vi "클러스터.vi"() -> ()   [LabVIEW 2014]
panel:
  out "클러스터 4":T1
  in  "클러스터 3":T1={"숫자형"=4.12, "확인 버튼"=TRUE, "문자열"="hello", "배열"=[1.0, -2.0, 3.0, -3.0, 7.5], "error in (no error)"={"status"=FALSE, "code"=0, "source"=""}}
  out "클러스터 2":T1
  in  "클러스터":T1={"숫자형"=4.12, "확인 버튼"=TRUE, "문자열"="hello", "배열"=[1.0, -2.0, 3.0, -3.0, 7.5], "error in (no error)"={"status"=FALSE, "code"=0, "source"=""}}
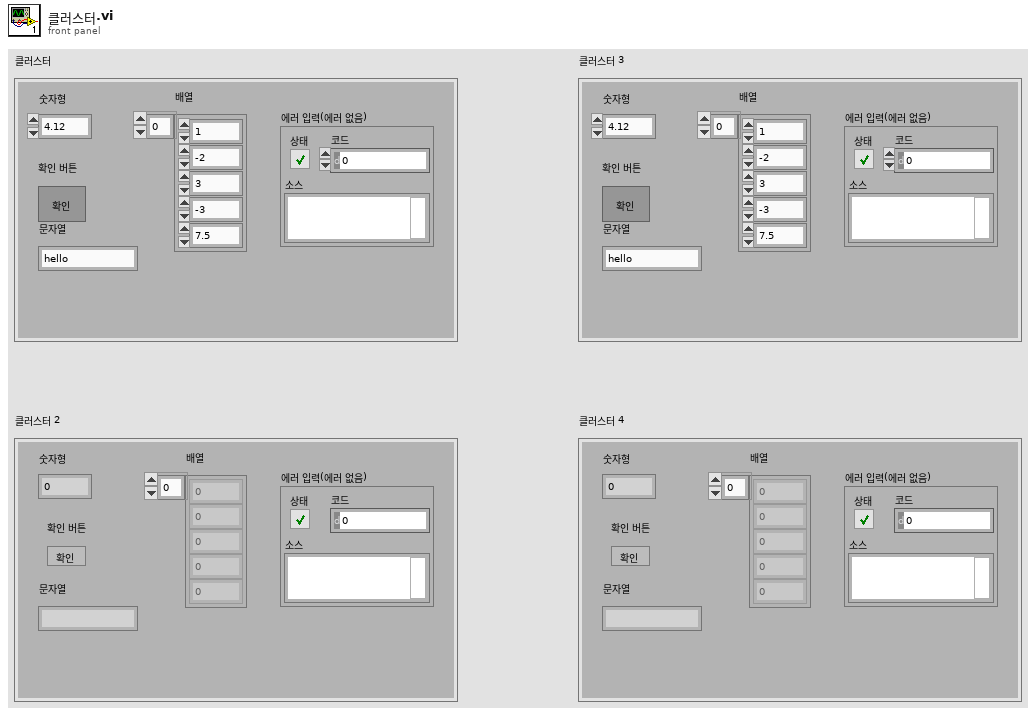
[diagram p1: front panel]
types:
  T1 = cluster{"숫자형":dbl, "확인 버튼":bool, "문자열":string, "배열":dbl[], "error in (no error)":errorcluster}
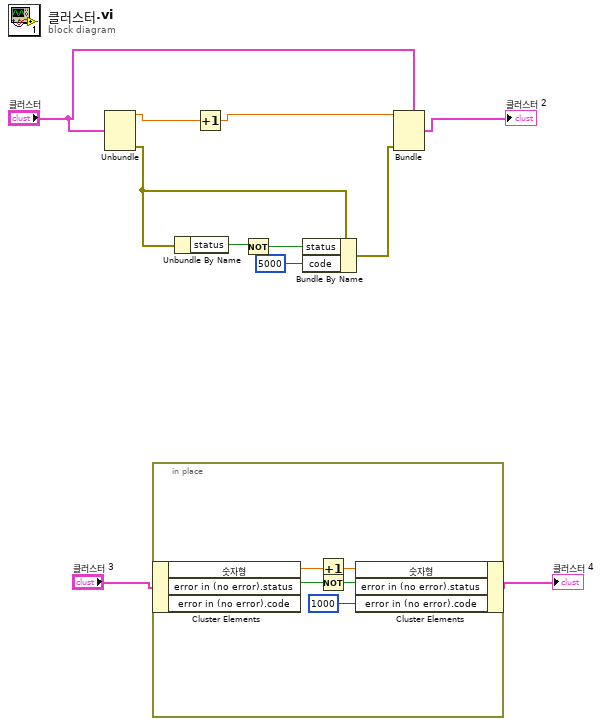
[diagram p0: block diagram]
diagram:
  n1 = Unbundle("클러스터") -> ("숫자형"=w10:dbl, "error in (no error)"=w7:errorcluster)  [unwired: 3 out]
  n2 = in-place {
    n3 = in-place-cluster #1("클러스터 3") -> ("숫자형"=w16:dbl, "error in (no error).status"=w14:bool)  [unwired: 1 out]
    n4 = Increment(x=w16) -> (x+1=w15:dbl)
    n5 = Not(x=w14) -> (.not. x?=w13:bool)
    n6 = in-place-cluster #1("숫자형"=w15, "error in (no error).status"=w13, "error in (no error).code"=1000) -> (→"클러스터 4":T1)
  }
  n7 = Unbundle By Name(w7) -> ("status"=w6:bool)
  n8 = Increment(x=w10) -> (x+1=w9:dbl)
  n9 = Not(x=w6) -> (.not. x?=w5:bool)
  n10 = Bundle By Name(cluster=w7, "status"=w5, "code"=5000) -> (w3:errorcluster)
  n11 = Bundle(cluster="클러스터", "숫자형"=w9, "error in (no error)"=w3) -> (→"클러스터 2":T1)  [unwired: 3 in]
